vi "Move Z Raster + B-Scan.vi"(0 "Reference In":refnum<class "_Controller.lvclass">, 1 "VISA resource name":refnum<visa-resource-name>, 2 "Source (0: Channel 1)":u16(ring) items=["Channel 1", "Channel 2", "Channel 3", "Channel 4", "Memory 1", "Memory 2", "Memory 3", "Memory 4", "Function 1", "Function 2", "Function 3", "Function 4", "Function 5", "Function 6", "Function 7", "Function 8"], 3 "Z Number of Steps":string="0", 4 "Initial Direction":bool=TRUE, 5 "Error In":errorcluster) -> (14 "Reference Out":refnum<class "_Controller.lvclass">, 16 "B-Scan":dbl[][](graph), 17 "A-Scan":waveform(dbl)[](graph), 19 "Error Out":errorcluster)   [LabVIEW 2020]
doc: "This incorporates both the motion of the machine as well as the reading from the oscilloscope in the Z direction. It then processes the incoming A-scan's mapping the values onto a B-scan. It automates the process of moving along the entire length of the Z desired length, stopping to scan at regular intervals and finally triggering the osciloscope at each scanning point and then the processing required for a B-scan.\n\nArgs:\n\nReference In: Incoming communication (reference) between LabView and the scanning rig controller\nError In: Checks for any errors with the incoming communication (reference)\nVISA Resource Name: Specifies the model of osciloscope being used \nSource (Channel): Specificies the channel that is being triggered for a reading\nZ Number of Steps: Number of steps to cover the entire Z length\nInitial Direction: Direction to move in the Z direction\n\nReturns:\n\nReference Out: Output communnication (reference) between LabView and controller\nError Out: Checks for any error with output communication (reference)\nB-Scan: Resultant B-scan from all the A-scan's along that axis\nA-Scan: A-scan in the form of a waveform, note it is within a for loop so outputs multiple A-scan's in this VI alone"
uses:
  <instrlib>/Arcus Ethernet Driver 1.0.0/ArcusEthernetComm/classes/Controller/_Controller.lvclass
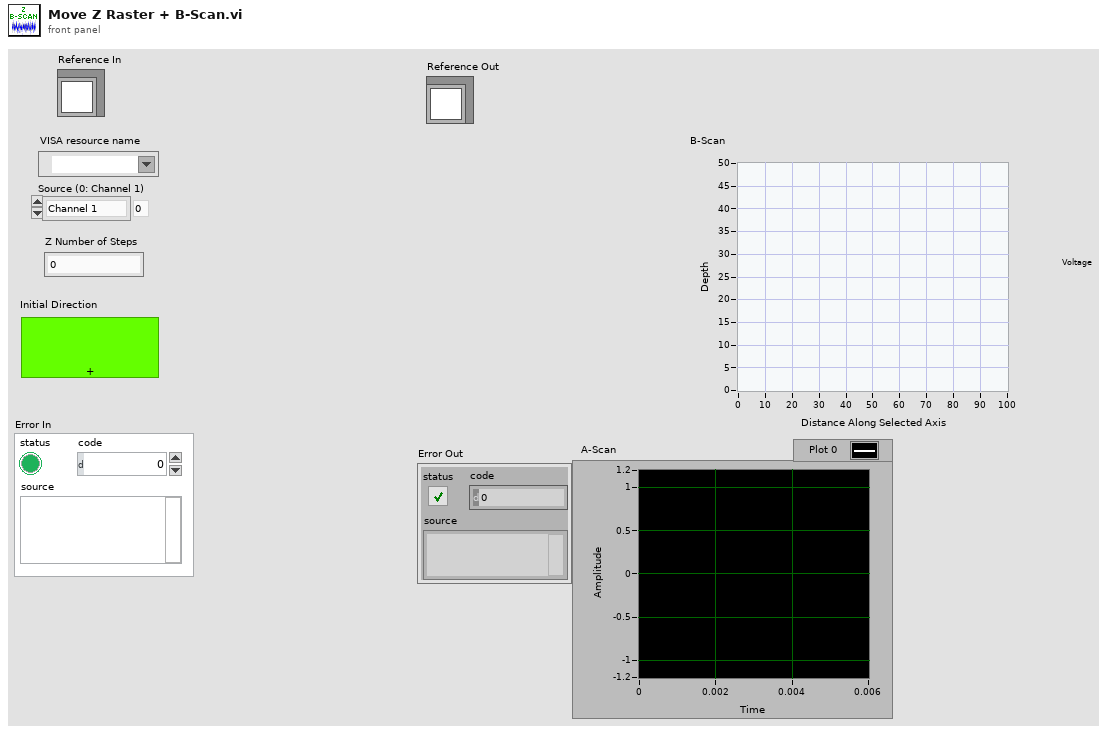
[diagram p1: front panel]
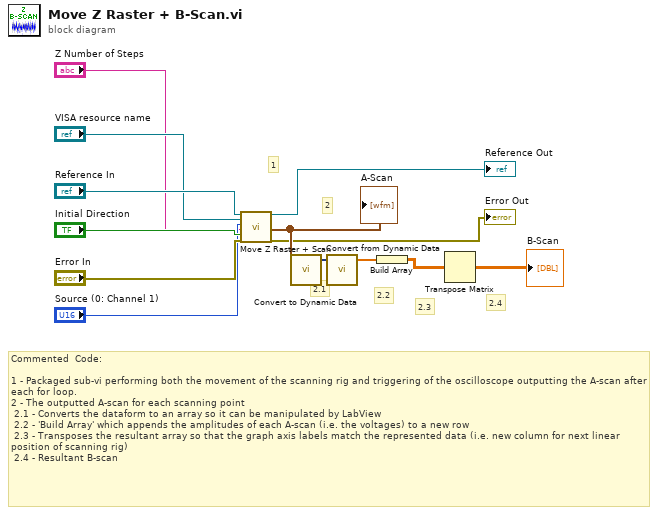
[diagram p0: block diagram]
diagram:
  # "2"
  # "2.3"
  # "2.4"
  # "2.2"
  # "2.1"
  # "1"
  # "Commented  Code: \n\n1 - Packaged sub-vi performing both the movement of the scanning rig and triggering of the oscilloscope outputting the A-scan after each for loop.\n2 - The outputted A-scan for each scanning point\n 2.1 - Converts the dataform to an array so it can be manipulated by LabView\n 2.2 - 'Build Array' which appends the amplitudes of each A-scan (i.e. the voltages) to a new row\n 2.3 - Transposes the resultant array so that the graph axis labels match the represented data (i.e. new column for next linear position of scanning rig)\n 2.4 - Resultant B-scan"
  n1 = call "Move Z Raster + Scan.vi"("Reference In"="Reference In", "VISA resource name"="VISA resource name", "Source (0: Channel 1)"="Source (0: Channel 1)", "Z Number of Steps"="Z Number of Steps", "Initial Direction"="Initial Direction", "Error In"="Error In") -> ("Reference Out"=→"Reference Out":refnum<class "_Controller.lvclass">, "A-Scan"=w3:waveform(dbl)[], "Error Out"=→"Error Out":errorcluster)  [unwired: 10 in, 1 out]
  "A-Scan" <- w3
  n2 = call "Convert to Dynamic Data"("Array of Waveforms"=w3) -> ("Dynamic Data Type"=w10:dynamicdata)  [unwired: 3 in]
  n3 = call "Convert from Dynamic Data"("Dynamic Data Type"=w10) -> ("Array"=w11:dbl[])  [unwired: 3 in]
  n4 = Build Array(w11) -> (w12:dbl[][])
  n5 = Transpose Matrix(1:w12) -> (0:→"B-Scan":dbl[][])
